vi "Analog Bank Write.vi"(8 "error in (no error)":errorcluster, 9 "Channels to set":i32[](array[numeric]), 10 "Values to set":sgl[](array[numeric]), 11 "TCP Network Connection in":refnum<k5>) -> (0 "error out":errorcluster, 3 "TCP Network Connection out":refnum<k5>)   [LabVIEW 2024, in "OptoMMP.lvlib"]
doc: "Performs an analog bank write on the specified TCP network. Writes the provided single-precision float values to the specified channels. \n\n\"Channels to set\" corresponds to points 0-63, for a total of 64 channels. Each module begins on the order of 4 points (module 0 starts at point 0, module 1 starts at point 4, etc.). \"Analog Bank Write\" must be preceded by \"OptoMMP Open Connection\".\n\nThe length of the \"Channels to set\" array must be equal to that of the \"Values to set\" array. Analog Bank Write can only be used with devices with firmware R9.4d or higher.\n\nLast updated: 8/6/2025"
uses:
  <instrlib>/OptoMMP/OptoMMP.lvlib
panel:
  # "Copyright (c) 2025 California Institute of Technology (Caltech).\nU.S. Government sponsorship acknowledged.\n\nLicensed under the Apache License, Version 2.0 (the \"License\");\nyou may not use this file except in compliance with the License.\nYou may obtain a copy of the License at\n\n    http://www.apache.org/licenses/LICENSE-2.0\n\nUnless required by applicable law or agreed to in writing, software\ndistributed under the License is distributed on an \"AS IS\" BASIS,\nWITHOUT WARRANTIES OR CONDITIONS OF ANY KIND, either express or implied.\nSee the License for the specific language governing permissions and\nlimitations under the License."
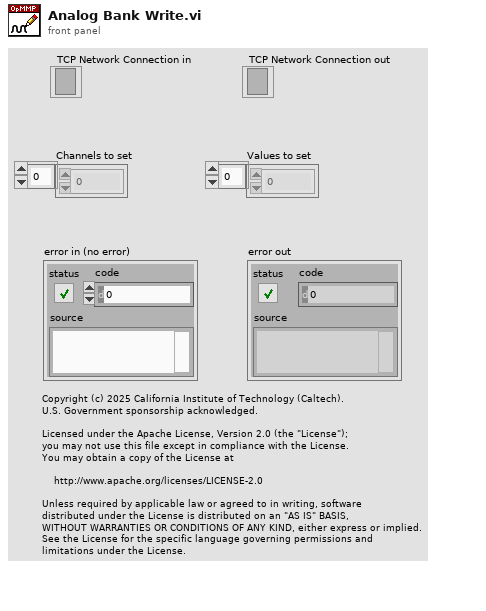
[diagram p1: front panel]
types:
  T1 = enum16{"Read Block Response", "Write Quadlet or Block Response", "Read Quadlet Response"}
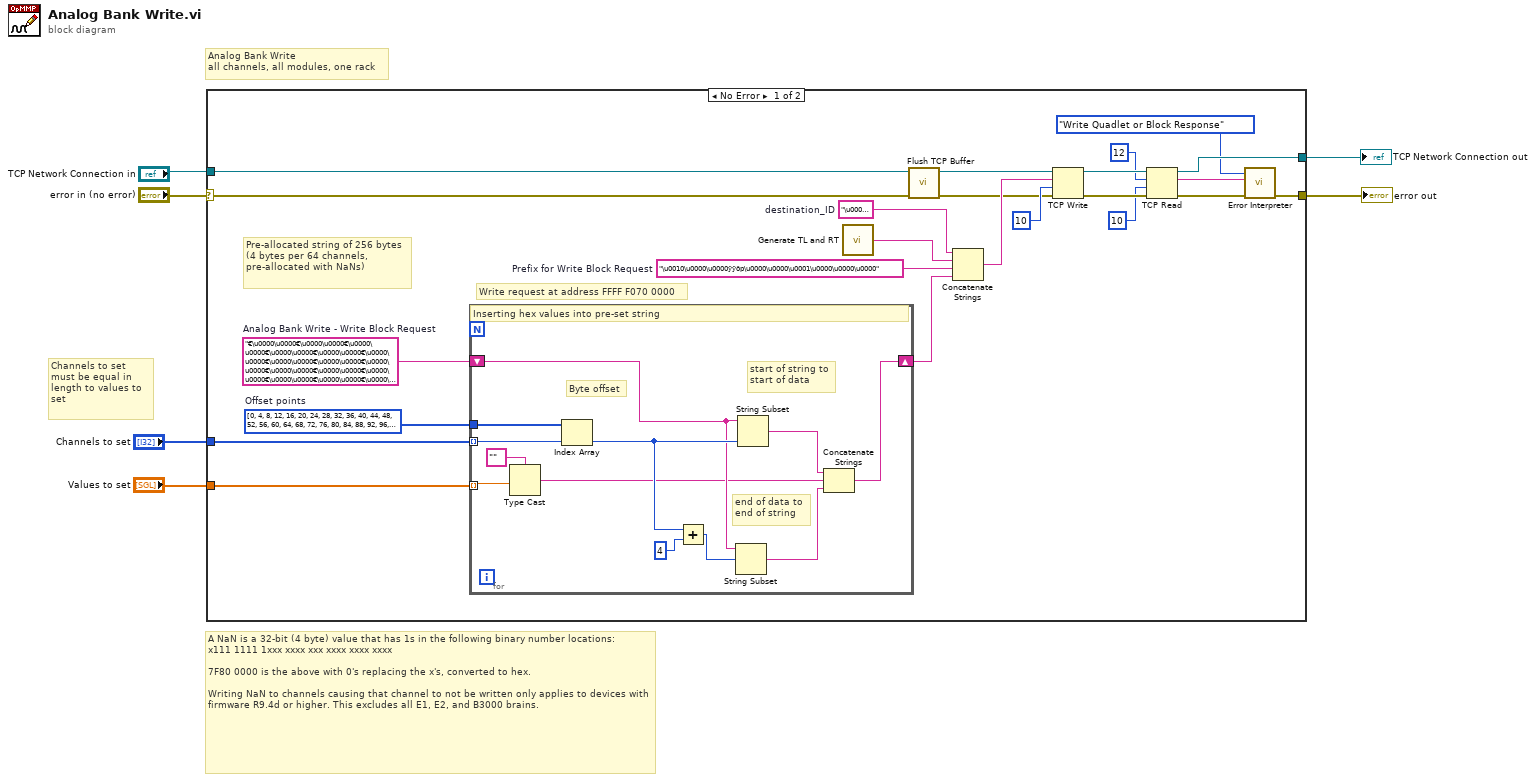
[diagram p0: block diagram]
diagram:
  # "Channels to set \nmust be equal in\nlength to values to \nset"
  # "Analog Bank Write\nall channels, all modules, one rack"
  # "A NaN is a 32-bit (4 byte) value that has 1s in the following binary number locations:\nx111 1111 1xxx xxxx xxx xxxx xxxx xxxx\n\n7F80 0000 is the above with 0's replacing the x's, converted to hex.\n\nWriting NaN to channels causing that channel to not be written only applies to devices with firmware R9.4d or higher. This excludes all E1, E2, and B3000 brains."
  n1 = case shown="No Error" "error in (no error)" {
    selector: "error in (no error)" -> [w12 w43]
    tunnel: "Values to set" -> [w29 _]
    tunnel: "Channels to set" -> [w28 _]
    tunnel: [w27 w43] -> w4
    tunnel: [w26 w42] -> w3
    tunnel: "TCP Network Connection in" -> [w13 w42]
    frame No Error {
      w7 = "\u0000\u0000"  # destination_ID
      w11 = "€\u0000\u0000€\u0000\u0000€\u0000\u0000€\u0000\u0000€\u0000\u0000€\u0000\u0000€\u0000\u0000€\u0000\u0000€\u0000\u0000€\u0000\u0000€\u0000\u0000€\u0000\u0000€\u0000\u0000€\u0000\u0000€\u0000\u0000€\u0000\u0000€\u0000\u0000€\u0000\u0000€\u0000\u0000€\u0000\u0000€\u0000\u0000€\u0000\u0000€\u0000\u0000€\u0000\u0000€\u0000\u0000€\u0000\u0000€\u0000\u0000€\u0000\u0000€\u0000\u0000€\u0000\u0000€\u0000\u0000€\u0000\u0000€\u0000\u0000€\u0000\u0000€\u0000\u0000€\u0000\u0000€\u0000\u0000€\u0000\u0000€\u0000\u0000€\u0000\u0000€\u0000\u0000€\u0000\u0000€\u0000\u0000€\u0000\u0000€\u0000\u0000€\u0000\u0000€\u0000\u0000€\u0000\u0000€\u0000\u0000€\u0000\u0000€\u0000\u0000€\u0000\u0000€\u0000\u0000€\u0000\u0000€\u0000\u0000€\u0000\u0000€\u0000\u0000€\u0000\u0000€\u0000\u0000€\u0000\u0000€\u0000\u0000€\u0000\u0000€\u0000\u0000€\u0000\u0000"  # Analog Bank Write - Write Block Request
      w10 = i32[] [0, 4, 8, 12, 16, 20, 24, 28, 32, 36, 40, 44, 48, 52, 56, 60, 64, 68, 72, 76, 80, 84, 88, 92, 96, 100, 104, 108, 112, 116, 120, 124, 128, 132, 136, 140, 144, 148, 152, 156, 160, 164, 168, 172, 176, 180, 184, 188, 192, 196, 200, 204, 208, 212, 216, 220, 224, 228, 232, 236, 240, 244, 248, 252]  # Offset points
      w23 = "\u0010\u0000\u0000ÿÿðp\u0000\u0000\u0001\u0000\u0000\u0000"  # Prefix for Write Block Request
      # "Pre-allocated string of 256 bytes  (4 bytes per 64 channels, pre-allocated with NaNs)"
      # "Write request at address FFFF F070 0000"
      n2 = for {
        tunnel: w28 -> [w39] mode=indexing
        tunnel: w29 -> [w41] mode=indexing
        shift-right: [w31] -> w25
        shift-left: w11 -> [w35]
        tunnel: w10 -> [w30]
        # "end of data to\nend of string"
        # "start of string to\nstart of data"
        # "Byte offset"
        # "Inserting hex values into pre-set string"
        n3 = Type Cast(type="", x=w41) -> (*(type *) &x=w32:string)
        n4 = Index Array(array=w30, index=w39) -> (element=w37:i32)
        n5 = Add(x=w37, y=4) -> (x+y=w36:i32)
        n6 = String Subset(string=w35, offset (0)=w36) -> (substring=w33:string)  [unwired: 1 in]
        n7 = String Subset(string=w35, length (rest)=w37) -> (substring=w34:string)  [unwired: 1 in]
        n8 = Concatenate Strings(w34, w32, w33) -> (w31:string)
      }
      n9 = call <instrlib>:"Generate TL and RT.vi"() -> ("tl + rt"=w8:string)
      n10 = call <instrlib>:"Flush TCP Buffer.vi"("error in (no error)"=w12, "TCP Network Connection in"=w13) -> ("error out"=w14:errorcluster, "TCP Network Connection out"=w15:refnum<k5>)  [unwired: 8 in]
      n11 = Concatenate Strings(w7, w8, w23, w25) -> (w24:string)
      n12 = TCP Write(connection ID=w15, data in=w24, error in (no error)=w14, 9:10 ("timeout ms (25000)")) -> (connection ID out=w21:refnum<k5>, error out=w20:errorcluster)  [unwired: 1 out]
      n13 = TCP Read(connection ID=w21, bytes to read=12, error in (no error)=w20, 9:10 ("timeout ms (25000)")) -> (connection ID out=w26:refnum<k5>, data out=w9:string, error out=w22:errorcluster)  [unwired: 1 in]
      n14 = call <instrlib>:"Error Interpreter.vi"("error in (no error)"=w22, "data in"=w9, "packet type"=T1."Write Quadlet or Block Response") -> ("error out"=w27:errorcluster)  [unwired: 8 in]
    }
    frame Error {
    }
  }
  "error out" <- w4
  "TCP Network Connection out" <- w3
